vi "readFlash.vi"(2 "bytesToRead":u16, 3 "offset":u32) -> (0 "return type":i32, 1 "buffer":u8[](array[numeric]))   [LabVIEW 2012]
uses:
  hidapi_32bits.dll
panel:
  out "string":string
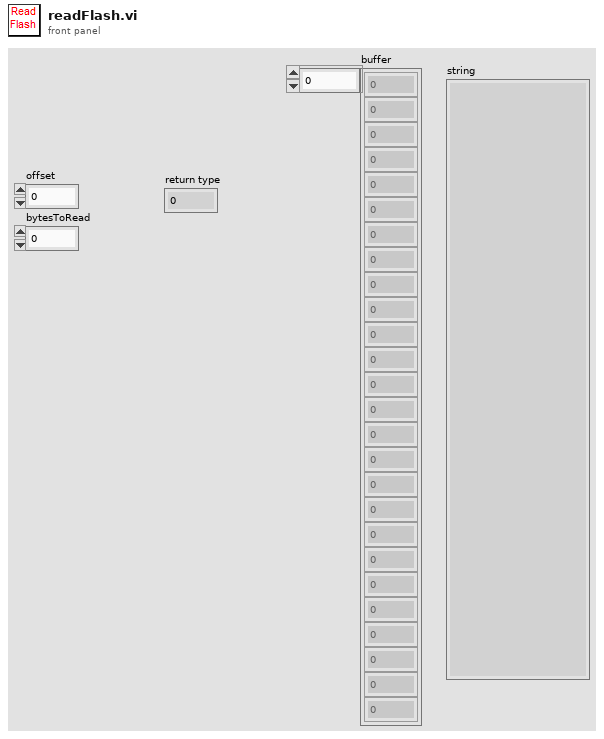
[diagram p1: front panel]
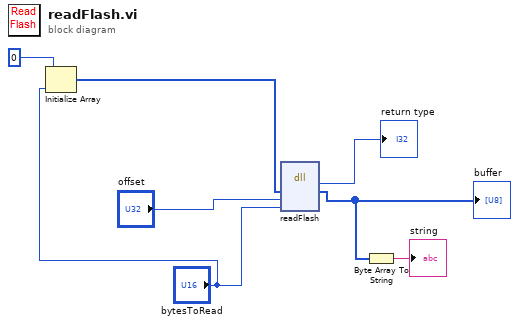
[diagram p0: block diagram]
diagram:
  n1 = Initialize Array(u8 0 ("element"), "bytesToRead") -> (w4:u8[])
  n2 = dll-call lib="C:/All_Data/mikrocont/Project1/New_controller__Jan_2015/LabView_Aug_2015/hidapi_32bits.dll" fn="readFlash"("buffer"=w4, "offset"="offset", "bytesToRead"="bytesToRead") -> ("return type"=→"return type":i32, "buffer"=w2:u8[])  [unwired: 5 in, 2 out]
  "buffer" <- w2
  n3 = Byte Array To String(unsigned byte array=w2) -> (string=→"string":string)
